vi "Read Device Name and Serial Number.vi"(8 "error in (no error)":errorcluster, 11 "Lotis in":refnum<class "PL Lotis TII LS.lvclass">) -> (0 "error out":errorcluster, 1 "serial number":string, 2 "name":string, 3 "Lotis out":refnum<class "PL Lotis TII LS.lvclass">)   [LabVIEW 2015, in "PL Lotis TII LS.lvclass"]
doc: "Reads device name and serial number."
uses:
  PL Lotis TII LS.lvclass
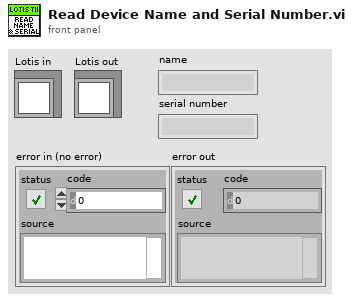
[diagram p1: front panel]
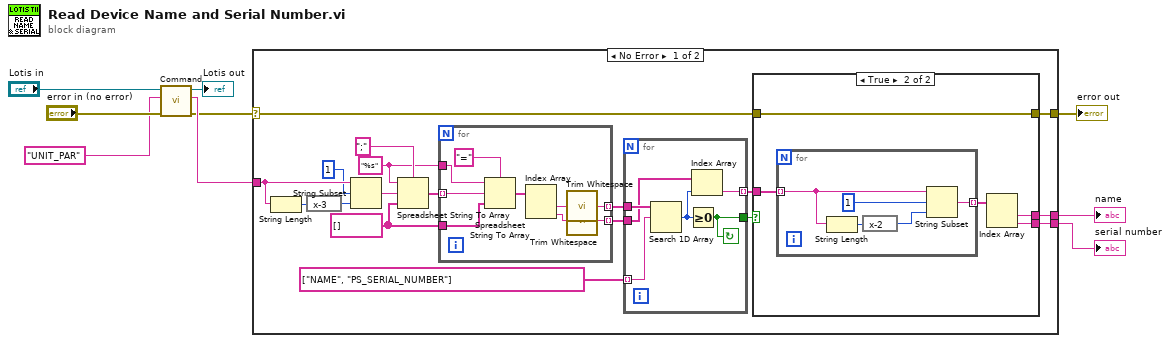
[diagram p0: block diagram]
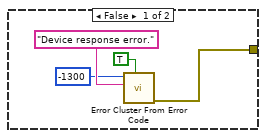
[diagram p2: hidden frame]
diagram:
  n1 = call "Command.vi"("error in (no error)"="error in (no error)", "command"="UNIT_PAR", "Lotis in"="Lotis in") -> ("error out"=w4:errorcluster, "response data"=w5:string, "Lotis out"=→"Lotis out":refnum<class "PL Lotis TII LS.lvclass">)  [unwired: 6 in]
  n2 = case shown="No Error" w4 {
    selector: w4 -> [w16 w57]
    tunnel: w5 -> [w27 _]
    tunnel: [w15 w57] -> w3
    tunnel: [w11 _] -> w2
    tunnel: [w10 _] -> w1
    frame No Error {
      w20 = "%s" ("format string")
      w19 = string[] [] ("array type (2D Dbl)")
      n3 = String Length(string=w27) -> (length=w25:i32)
      n4 = expression code="x-3"(w25) -> (w24:i32)
      n5 = String Subset(string=w27, offset (0)=1, length (rest)=w24) -> (substring=w23:string)
      n6 = Spreadsheet String To Array(delimiter (Tab)=";", format string=w20, spreadsheet string=w23, array type (2D Dbl)=w19) -> (array=w21:string[])
      n7 = for {
        tunnel: w21 -> [w53] mode=indexing
        tunnel: w20 -> [w56]
        tunnel: w19 -> [w54]
        tunnel: [w49] -> w18 mode=indexing
        tunnel: [w48] -> w13 mode=indexing
        n8 = Spreadsheet String To Array(delimiter (Tab)="=", format string=w56, spreadsheet string=w53, array type (2D Dbl)=w54) -> (array=w52:string[])
        n9 = Index Array(array=w52) -> (element #1=w51:string, element #2=w50:string)  [unwired: 2 in]
        n10 = call <vilib>:"Trim Whitespace.vi"("string"=w51) -> ("trimmed string"=w49:string)  [unwired: 1 in]
        n11 = call <vilib>:"Trim Whitespace.vi"("string"=w50) -> ("trimmed string"=w48:string)  [unwired: 1 in]
      }
      n12 = for {
        tunnel: w18 -> [w47]
        tunnel: string[] ["NAME", "PS_SERIAL_NUMBER"] -> [w46] mode=indexing
        tunnel: [w45] -> w14
        tunnel: w13 -> [w44]
        tunnel: [w42] -> w12 mode=indexing
        stop <- w45 continue-if-true
        n13 = Search 1D Array(1D array=w47, element=w46) -> (index of element=w43:i32)  [unwired: 1 in]
        n14 = Greater Or Equal To 0?(x=w43) -> (x >= 0?=w45:bool)
        n15 = Index Array(array=w44, index=w43) -> (element=w42:string)
      }
      n16 = case shown="True" w14 {
        tunnel: w16 -> [_ w36]
        tunnel: [w28 w36] -> w15
        tunnel: w12 -> [_ w35]
        tunnel: [_ w33] -> w11
        tunnel: [_ w32] -> w10
        frame False {
          n17 = call <vilib>:"Error Cluster From Error Code.vi"("show call chain? (False)"=TRUE, "error message (\"\")"="Device response error." ("format string"), "error code (0)"=-1300) -> ("error out"=w28:errorcluster)  [unwired: 6 in]
        }
        frame True {
          n18 = for {
            tunnel: w35 -> [w38] mode=indexing
            tunnel: [w37] -> w34 mode=indexing
            n19 = String Length(string=w38) -> (length=w40:i32)
            n20 = expression code="x-2"(w40) -> (w39:i32)
            n21 = String Subset(string=w38, offset (0)=1, length (rest)=w39) -> (substring=w37:string)
          }
          n22 = Index Array(array=w34) -> (element #1=w33:string, element #2=w32:string)  [unwired: 2 in]
        }
      }
    }
    frame Error {
    }
  }
  "error out" <- w3
  "name" <- w2
  "serial number" <- w1
